vi "Calculate Next Value Index.vi"(10 "message":T1={"name"="", "message type"="BC to RT", "endpoint Rx"={"terminal address"=0, "subaddress"=0}, "endpoint Tx"={"terminal address"=0, "subaddress"=0}, "mode code"=0, "number of words"=0, "parameters"=[], "create timestamp channel"=FALSE}, 11 "value index":i32) -> (3 "next value index":i32)   [LabVIEW 2020, in "Ballard MIL-STD-1553 Engine.lvlib" / "Custom Device.lvlib"]
uses:
  Custom Device.lvlib
  Shared/Address.ctl
  Shared/Terminal Endpoint.ctl
  Shared/Parameter Definition.ctl
  Shared/Message Type.ctl
  Shared/Message Definition.ctl
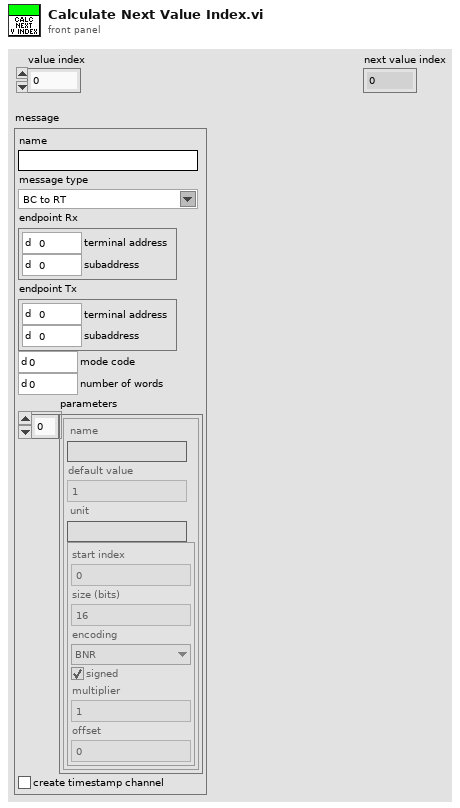
[diagram p1: front panel]
types:
  T1 = typedef "Message Definition.ctl" = cluster{"name":string, "message type":T2, "endpoint Rx":T3, "endpoint Tx":T3, "mode code":u16, "number of words":u16, "parameters":cluster{"name":string, "default value":dbl, "unit":string, "parameter definition":T5}[], "create timestamp channel":bool}
  T2 = typedef "Message Type.ctl" = string
  T3 = typedef "Terminal Endpoint.ctl" = cluster{"terminal address":T4, "subaddress":T4}
  T4 = typedef "Address.ctl" = u16
  T5 = typedef "Parameter Definition.ctl" = cluster{"start index":i32, "size (bits)":i32, "encoding":enum16{"BNR", "BCD", "Discrete"}, "signed":bool, "multiplier":dbl, "offset":dbl}
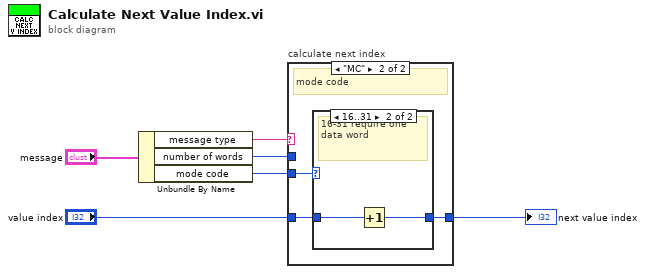
[diagram p0: block diagram]
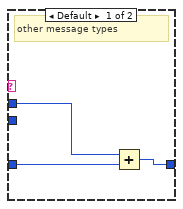
[diagram p2: hidden frame]
diagram:
  n1 = Unbundle By Name("message") -> ("message type"=w4:T2, "number of words"=w5:u16, "mode code"=w6:u16)
  n2 = case "calculate next index" shown="\"MC\"" w4 {
    tunnel: [w7 w11] -> w1
    tunnel: "value index" -> [w9 w12]
    tunnel: w5 -> [w8 _]
    tunnel: w6 -> [_ w10]
    frame Default {
      # "other message types"
      n3 = Add(x=w8, y=w9) -> (x+y=w7:i32)
    }
    frame "MC" {
      # "mode code"
      n4 = case shown="16..31" w10 {
        tunnel: w12 -> [w13 w15]
        tunnel: [w13 w14] -> w11
        frame 0, Default {
          # "0-15 require no data word"
        }
        frame 16..31 {
          # "16-31 require one data word"
          n5 = Increment(x=w15) -> (x+1=w14:i32)
        }
      }
    }
  }
  "next value index" <- w1
